vi "ImageNotifyGen.vi"() -> (0 "ImageClusterref":T1, 1 "ImageNotify":refnum<notifier>)   [LabVIEW 2012]
panel:
  in  "ImageCluster":T1
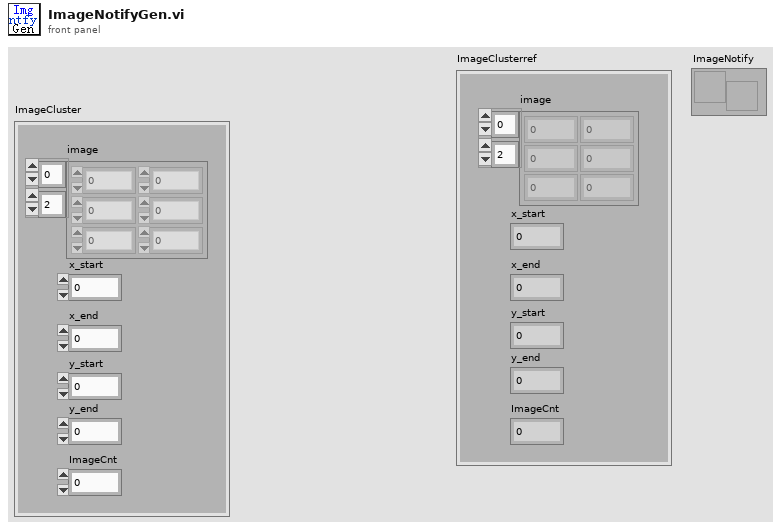
[diagram p1: front panel]
types:
  T1 = cluster{"image":i16[][], "x_start":u32, "x_end":u32, "y_start":u32, "y_end":u32, "ImageCnt":u32}
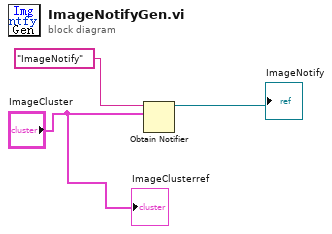
[diagram p0: block diagram]
diagram:
  n1 = Obtain Notifier(name (unnamed)="ImageNotify" ("名称（未命名）"), notification data type="ImageCluster") -> (notifier out=→"ImageNotify":refnum<notifier>)  [unwired: 2 in, 2 out]
  "ImageClusterref" <- "ImageCluster"
